vi "Prompt user - load & display.vi"(7 "Image space":T1, 8 "error in (no error)":errorcluster, 11 "Start path":path) -> (0 "error out":errorcluster, 2 "name":string, 5 "Image Out":T1)   [LabVIEW 2013]
doc: "Asks the user to select an image, loads the image into display image and draws the imaq window.\n\nNote - the displayed image is compressed by the display factor."
uses:
  <vilib>/vision/Image Controls.llb/IMAQ Image.ctl
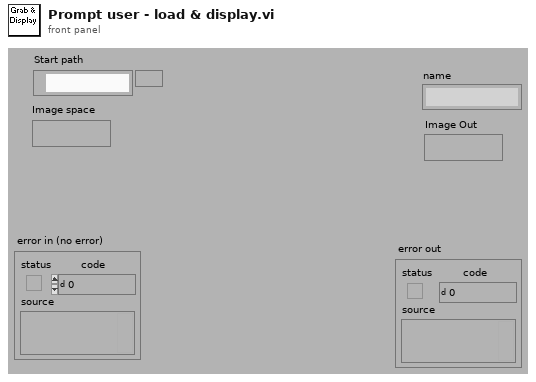
[diagram p1: front panel]
types:
  T1 = typedef "IMAQ Image.ctl" = refnum<image>
  T2 = enum32{"existing file", "new file", "new or existing file", "existing dir", "new dir", "new or existing dir", "existing file (use LLBs)", "new file (use LLBs)", "new or existing file (use LLBs)", "new or existing file or directory (use LLBs)"}
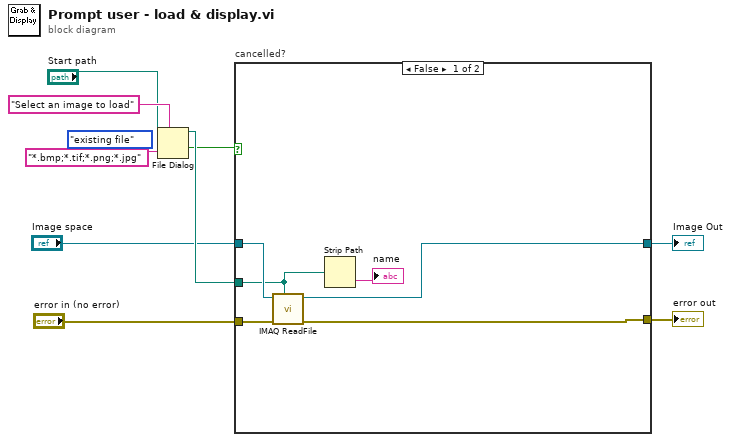
[diagram p0: block diagram]
diagram:
  (unwired) T2."existing file" ("select mode (2)")
  n1 = File Dialog(6:"*.bmp;*.tif;*.png;*.jpg" ("pattern"), 7:"Select an image to load" ("prompt"), 11:"Start path") -> (1:w5:bool, 3:w6:path)  [unwired: 4 in, 2 out]
  n2 = case "cancelled?" shown="False" w5 {
    tunnel: [w12 w17] -> w9
    tunnel: w6 -> [w13 _]
    tunnel: "Image space" -> [w15 w16]
    tunnel: "error in (no error)" -> [w14 w17]
    tunnel: [w10 w16] -> w1
    frame False {
      n3 = call "IMAQ ReadFile"("File Path"=w13, "error in (no error)"=w14, "Image"=w15) -> ("error out"=w12:errorcluster, "Image Out"=w10:T1)  [unwired: 4 in, 3 out]
      n4 = Strip Path(path=w13) -> (name=→"name":string)  [unwired: 1 out]
    }
    frame True {
    }
  }
  "error out" <- w9
  "Image Out" <- w1
